vi "WriteAO.vi"(8 "error in":errorcluster, 9 "PWM Settings":T1 {"Frequency" format="%#pHz"; "Duty" format="%.02f%%"}, 10 "Analog Output":T2, 11 "VISA resource name":refnum<visa-resource-name>) -> (0 "error out":errorcluster, 3 "VISA resource name out":refnum<visa-resource-name>)   [LabVIEW 2020, in "HandsOnPi2040.lvlib"]
doc: "Establishes communication with the instrument and optionally performs an instrument identification query and/or an instrument reset. It also places the instrument in a default state needed for other instrument driver operations. Therefore, call this VI before calling other instrument driver VIs for this instrument. Generally, you need to call the <b>Initialize</b> VI only once at the beginning of an application."
uses:
  HandsOnPi2040.lvlib
  AOs.ctl
  PWMSettings.ctl
  <vilib>/CTI/CTI Visa Drivers/CTI-Visa/CTI-Visa.lvlib
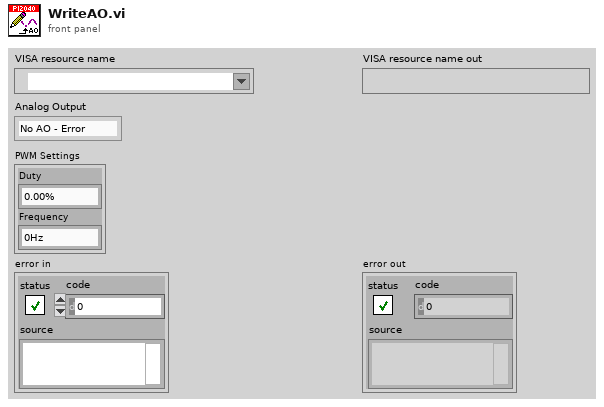
[diagram p1: front panel]
types:
  T1 = typedef "HandsOnPi2040.lvlib/PWMSettings.ctl" = cluster{"Duty":sgl, "Frequency":sgl}
  T2 = typedef "HandsOnPi2040.lvlib/AOs.ctl" = enum8{"No AO - Error", "AO1 (GPIO28)"}
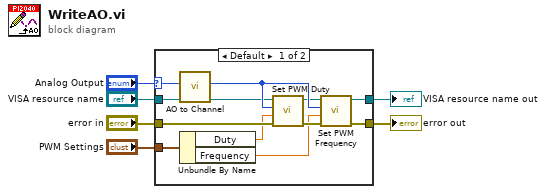
[diagram p0: block diagram]
diagram:
  n1 = case shown="Default" "Analog Output" {
    selector: "Analog Output" -> [w7 _]
    tunnel: [w17 w19] -> w5
    tunnel: [w11 w18] -> w4
    tunnel: "VISA resource name" -> [w13 w18]
    tunnel: "error in" -> [w16 w19]
    tunnel: "PWM Settings" -> [w8 _]
    frame Default {
      n2 = call "AO to Channel.vi"("Analog Output"=w7) -> ("Channel"=w14:i32)  [unwired: 10 in]
      n3 = Unbundle By Name(w8) -> ("Duty"=w10:sgl, "Frequency"=w9:sgl)
      n4 = call <vilib>:"Set PWM Duty.vi"("error in (no error)"=w16, "Duty % (0-1)"=w10, "Channel"=w14, "VISA resource name in"=w13) -> ("error out"=w15:errorcluster, "VISA resource name"=w12:refnum<visa-resource-name>)  [unwired: 6 in]
      n5 = call <vilib>:"Set PWM Frequency.vi"("error in (no error)"=w15, "Freq Hz"=w9, "Channel"=w14, "VISA resource name in"=w12) -> ("error out"=w17:errorcluster, "VISA resource name"=w11:refnum<visa-resource-name>)  [unwired: 6 in]
    }
    frame "No AO - Error" {
    }
  }
  "VISA resource name out" <- w4
  "error out" <- w5
